vi "get_installer_locations.vi"(8 "error in (no error)":errorcluster) -> (0 "error out":errorcluster, 3 "path []":path[](array[path]))   [LabVIEW 2015, in "lv-post-installer.lvlib"]
uses:
  lv-post-installer.lvlib
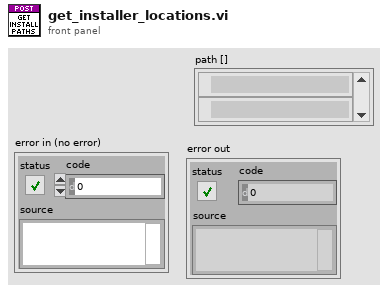
[diagram p1: front panel]
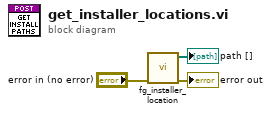
[diagram p0: block diagram]
diagram:
  n1 = call "fg_installer_location.vi"("error in (no error)"="error in (no error)") -> ("error out"=→"error out":errorcluster, "path [] out"=→"path []":path[])  [unwired: 9 in]
